vi "ProcessGObjectAsCallLibrary.vi"(8 "error in":errorcluster, 11 "GObject Ref":refnum<vi>) -> (0 "error out":errorcluster, 2 "Is SDL?":bool, 3 "GObject Ref As Call Library":refnum<vi>)   [LabVIEW 2024, in "CustomActions.lvlib"]
uses:
  CustomActions.lvlib
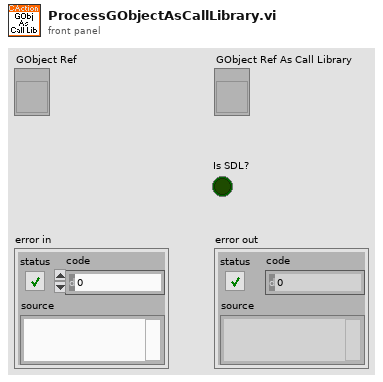
[diagram p1: front panel]
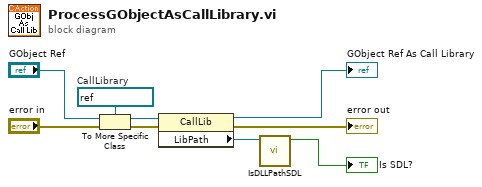
[diagram p0: block diagram]
diagram:
  w9 = refnum<vi> refnum  # CallLibrary
  n1 = To More Specific Class(target class=w9, reference="GObject Ref", error in="error in") -> (specific class reference=w7:refnum<vi>, error out=w8:errorcluster)
  n2 = property class="CallLib"(reference=w7, error in=w8) -> (reference out=→"GObject Ref As Call Library":refnum<vi>, error out=→"error out":errorcluster, "LibPath"=w6:path)
  n3 = call "IsDLLPathSDL.vi"("DLL Path"=w6) -> ("Is SDL?"=→"Is SDL?":bool)  [unwired: 7 in, 3 out]
